vi "Find Window.vi"(8 "error in (no error)":errorcluster, 11 "Window Name":string) -> (0 "error out":errorcluster, 3 "Win32 Window Handle":i32)   [LabVIEW 2020]
doc: "This VI calls the FindWindows Function in the User32.dll to obtain the Win32 Window handle for the Window specified by Window Name."
uses:
  kernel32.dll
  user32.dll
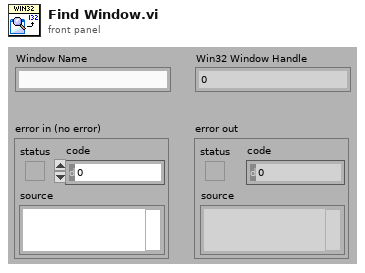
[diagram p1: front panel]
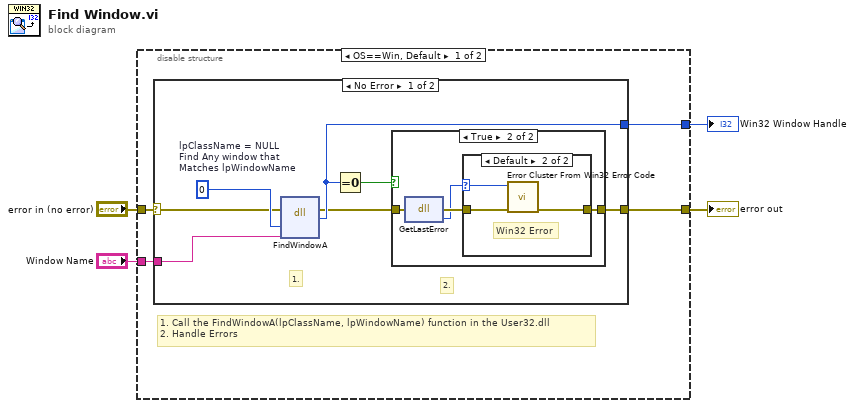
[diagram p0: block diagram]
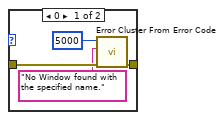
[diagram p3: hidden frame]
diagram:
  n1 = disable-structure shown="OS==Win, Default" {
    disable-tunnel: "Window Name" -> [w8 _]
    disable-tunnel: [w7 _] -> w3
    disable-tunnel: [w6 w29] -> w2
    disable-tunnel: "error in (no error)" -> [w5 w29]
    frame condition #0 (active) {
      # "1. Call the FindWindowA(lpClassName, lpWindowName) function in the User32.dll\n2. Handle Errors"
      n2 = case shown="No Error" w5 {
        selector: w5 -> [w11 w28]
        tunnel: w8 -> [w14 _]
        tunnel: [w13 _] -> w7
        tunnel: [w12 w28] -> w6
        frame No Error {
          w15 = u32 0  # lpClassName = NULL Find Any window that Matches lpWindowName
          # "2."
          # "1."
          n3 = dll-call lib="user32.dll" fn="FindWindowA"(error in=w11, "lpClassName"=w15, "lpWindowName"=w14) -> (error out=w9:errorcluster, "return type"=w13:i32)  [unwired: 4 in, 1 out]
          n4 = Equal To 0?(x=w13) -> (x = 0?=w10:bool)
          n5 = case shown="True" w10 {
            tunnel: [w16 w20] -> w12
            tunnel: w9 -> [w16 w19]
            frame False {
            }
            frame True {
              n6 = dll-call lib="kernel32.dll" fn="GetLastError" ("user32.dll:FindWindowA")(error in=w19) -> (error out=w18:errorcluster, "return type"=w17:i32)  [unwired: 2 in, 1 out]
              n7 = case shown="Default" w17 {
                selector: w17 -> [_ w25]
                tunnel: [w24 w27] -> w20
                tunnel: w18 -> [w23 w26]
                frame 0 {
                  n8 = call <vilib>:"Error Cluster From Error Code.vi"("error in (no error)"=w23, "error message (\"\")"="No Window found with the specified name." ("error message (\"\")"), "error code (0)"=5000) -> ("error out"=w24:errorcluster)  [unwired: 1 in, 5 out]
                }
                frame Default {
                  # "Win32 Error"
                  n9 = call "Error Cluster From Win32 Error Code.vi"("error in (no error)"=w26, "error code (0)"=w25) -> ("error out"=w27:errorcluster)  [unwired: 2 in, 7 out]
                }
              }
            }
          }
        }
        frame Error {
        }
      }
    }
    frame condition #1 {
    }
  }
  "error out" <- w2
  "Win32 Window Handle" <- w3
